vi "FeedbackDecode_KalmanMvnts2Str.vi"(1 "KMvntClust":T1={"KGain"=[[1.0, 1.0, -1.0, 1.0], [1.0, 1.0, -1.0, 1.0], [1.0, 1.0, -1.0, 1.0], [1.0, 1.0, -1.0, 1.0], [1.0, 1.0, -1.0, 1.0], [1.0, 1.0, -1.0, 1.0], [1.0, 1.0, -1.0, 1.0], [1.0, 1.0, -1.0, 1.0], [1.0, 1.0, -1.0, 1.0], [1.0, 1.0, -1.0, 1.0], [1.0, 1.0, -1.0, 1.0], [1.0, 1.0, -1.0, 1.0]], "KMvnts"={"Thumb"=FALSE, "Index"=FALSE, "Middle"=FALSE, "Ring"=FALSE, "Little"=FALSE, "ThumbInt"=FALSE, "IndexInt"=FALSE, "RingInt"=FALSE, "LittleInt"=FALSE, "WristPitch"=FALSE, "WristYaw"=FALSE, "WristRoll"=FALSE}, "KThresh"=[[0.2, 0.2, -1.0, 1.0], [0.2, 0.2, -1.0, 1.0], [0.2, 0.2, -1.0, 1.0], [0.2, 0.2, -1.0, 1.0], [0.2, 0.2, -1.0, 1.0], [0.2, 0.2, -1.0, 1.0], [0.2, 0.2, -1.0, 1.0], [0.2, 0.2, -1.0, 1.0], [0.2, 0.2, -1.0, 1.0], [0.2, 0.2, -1.0, 1.0], [0.2, 0.2, -1.0, 1.0], [0.2, 0.2, -1.0, 1.0]], "CtrlMode"=[enum."Position", enum."Position", enum."Position", enum."Position", enum."Position", enum."Position", enum."Position", enum."Position", enum."Position", enum."Position", enum."Position", enum."Position"], "CtrlSpd"=[1.0, 1.0, 1.0, 1.0, 1.0, 1.0, 1.0, 1.0, 1.0, 1.0, 1.0, 1.0]} {"CtrlSpd" min=0 max=1; "KThresh" min=0 max=1; "KGain" min=0}) -> (0 "KMvntStr":string)   [LabVIEW 2020]
panel:
  # "DOF"
  # "Gain (F/E)"
  # "Thresh (F/E)"
  # "Mode"
  # "Spd"
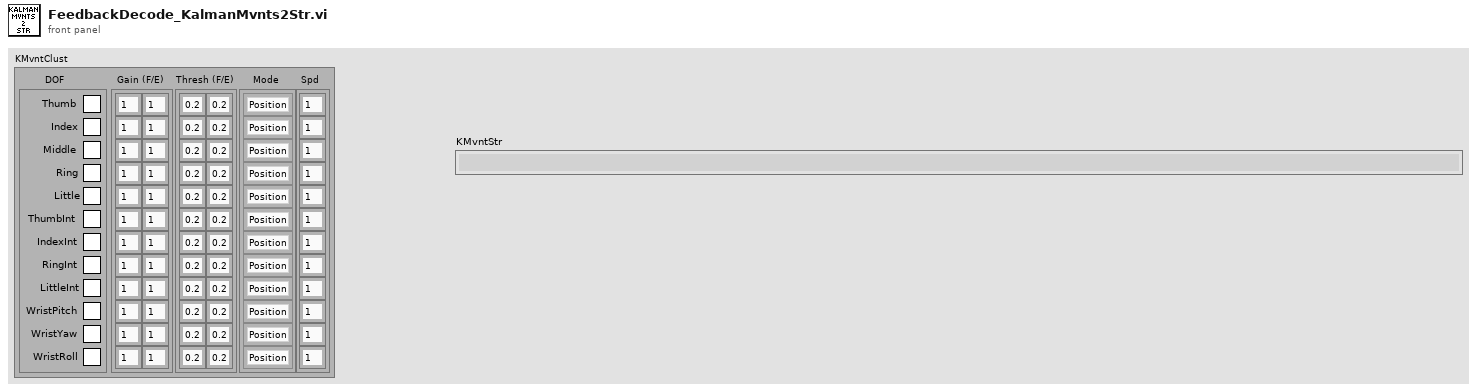
[diagram p1: front panel]
types:
  T1 = cluster{"KGain":sgl[][], "KMvnts":cluster{"Thumb":bool, "Index":bool, "Middle":bool, "Ring":bool, "Little":bool, "ThumbInt":bool, "IndexInt":bool, "RingInt":bool, "LittleInt":bool, "WristPitch":bool, "WristYaw":bool, "WristRoll":bool}, "KThresh":sgl[][], "CtrlMode":enum16{"Position", "Latching", "Leaky", "Velocity"}[], "CtrlSpd":sgl[]}
  T2 = cluster{"Thumb":bool, "Index":bool, "Middle":bool, "Ring":bool, "Little":bool, "ThumbInt":bool, "IndexInt":bool, "RingInt":bool, "LittleInt":bool, "WristPitch":bool, "WristYaw":bool, "WristRoll":bool}
  T3 = enum16{"Position", "Latching", "Leaky", "Velocity"}[]
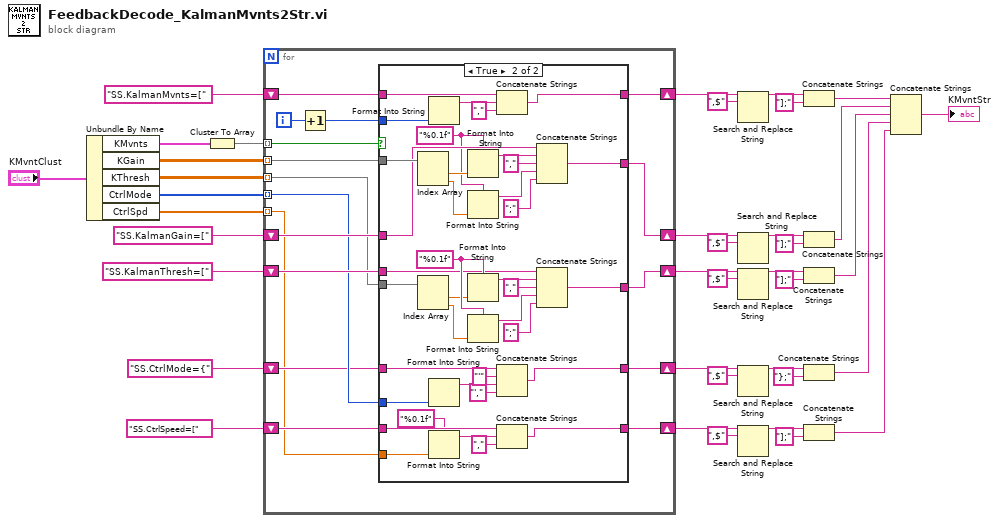
[diagram p0: block diagram]
diagram:
  n1 = Unbundle By Name("KMvntClust") -> ("KMvnts"=w15:T2, "KGain"=w32:sgl[][], "KThresh"=w23:sgl[][], "CtrlMode"=w14:T3, "CtrlSpd"=w7:sgl[])
  n2 = Cluster To Array(cluster=w15) -> (array=w16:bool[])
  n3 = for {
    shift-right: [w54] -> w35
    shift-left: "SS.KalmanMvnts=[" ("string") -> [w55]
    tunnel: w16 -> [w52] mode=indexing
    tunnel: w32 -> [w51] mode=indexing
    shift-right: [w50] -> w28
    shift-left: "SS.KalmanGain=[" ("string") -> [w49]
    shift-right: [w46] -> w19
    shift-left: "SS.KalmanThresh=[" ("string") -> [w48]
    tunnel: w23 -> [w47] mode=indexing
    tunnel: w14 -> [w44] mode=indexing
    shift-right: [w42] -> w9
    shift-left: "SS.CtrlMode={" ("string") -> [w43]
    tunnel: w7 -> [w40] mode=indexing
    shift-right: [w39] -> w2
    shift-left: "SS.CtrlSpeed=[" ("string") -> [w41]
    i -> [w53]
    n4 = Increment(x=w53) -> (x+1=w45:i32)
    n5 = case shown="True" w52 {
      tunnel: w55 -> [w60 w97]
      tunnel: [w60 w96] -> w54
      tunnel: w45 -> [_ w93]
      tunnel: w51 -> [_ w92]
      tunnel: [w59 w85] -> w50
      tunnel: w49 -> [w59 w84]
      tunnel: w48 -> [w58 w75]
      tunnel: w47 -> [_ w74]
      tunnel: [w58 w73] -> w46
      tunnel: w44 -> [_ w70]
      tunnel: w43 -> [w57 w69]
      tunnel: [w57 w67] -> w42
      tunnel: w41 -> [w56 w64]
      tunnel: w40 -> [_ w63]
      tunnel: [w56 w61] -> w39
      frame False {
      }
      frame True {
        w82 = "%0.1f" ("format string")
        w83 = "%0.1f" ("format string")
        n6 = Index Array(array=w92) -> (element #1=w91:sgl, element #2=w90:sgl)  [unwired: 2 in]
        n7 = Index Array(array=w74) -> (element #1=w76:sgl, element #2=w77:sgl)  [unwired: 2 in]
        n8 = Format Into String(w93) -> (resulting string=w95:string)  [unwired: 3 in, 1 out]
        n9 = Format Into String(w70) -> (resulting string=w71:string)  [unwired: 3 in, 1 out]
        n10 = Format Into String(format string="%0.1f", w63) -> (resulting string=w65:string)  [unwired: 2 in, 1 out]
        n11 = Format Into String(format string=w83, w91) -> (resulting string=w89:string)  [unwired: 2 in, 1 out]
        n12 = Format Into String(format string=w83, w90) -> (resulting string=w87:string)  [unwired: 2 in, 1 out]
        n13 = Format Into String(format string=w82, w76) -> (resulting string=w78:string)  [unwired: 2 in, 1 out]
        n14 = Format Into String(format string=w82, w77) -> (resulting string=w80:string)  [unwired: 2 in, 1 out]
        n15 = Concatenate Strings(w97, w95, "," ("string")) -> (w96:string)
        n16 = Concatenate Strings(w69, "'" ("string"), w71, "'," ("string")) -> (w67:string)
        n17 = Concatenate Strings(w64, w65, "," ("string")) -> (w61:string)
        n18 = Concatenate Strings(w84, w89, "," ("string"), w87, ";" ("string")) -> (w85:string)
        n19 = Concatenate Strings(w75, w78, "," ("string"), w80, ";" ("string")) -> (w73:string)
      }
    }
  }
  n20 = Search and Replace String(input string=w35, search string=",$") -> (result string=w37:string)  [unwired: 6 in, 3 out]
  n21 = Search and Replace String(input string=w28, search string=",$") -> (result string=w30:string)  [unwired: 6 in, 3 out]
  n22 = Search and Replace String(input string=w19, search string=",$") -> (result string=w21:string)  [unwired: 6 in, 3 out]
  n23 = Search and Replace String(input string=w9, search string=",$") -> (result string=w11:string)  [unwired: 6 in, 3 out]
  n24 = Search and Replace String(input string=w2, search string=",$") -> (result string=w4:string)  [unwired: 6 in, 3 out]
  n25 = Concatenate Strings(w37, "];" ("string")) -> (w27:string)
  n26 = Concatenate Strings(w30, "];" ("string")) -> (w26:string)
  n27 = Concatenate Strings(w21, "];" ("string")) -> (w18:string)
  n28 = Concatenate Strings(w11, "};" ("string")) -> (w8:string)
  n29 = Concatenate Strings(w4, "];" ("string")) -> (w1:string)
  n30 = Concatenate Strings(w27, w26, w18, w8, w1) -> (→"KMvntStr":string)
